vi "test_CCD_Setup_Testenvironment.vi"(6 "Delay between send and receive [ms]":i32=100, 8 "error in":errorcluster) -> (0 "error out":errorcluster, 2 "device open for communication?":bool, 3 "CCD out":refnum<class "CCD.lvclass">, 4 "Module Was Already Running?":bool)   [LabVIEW 2023]
uses:
  Classes/CCD/CCD.lvclass
  Libraries/DeviceManager/DeviceManager.lvlib
  <userlib>/_OpenG.lib/error/error.llb/openg_error.lvlib
panel:
  # "Connector Pane"
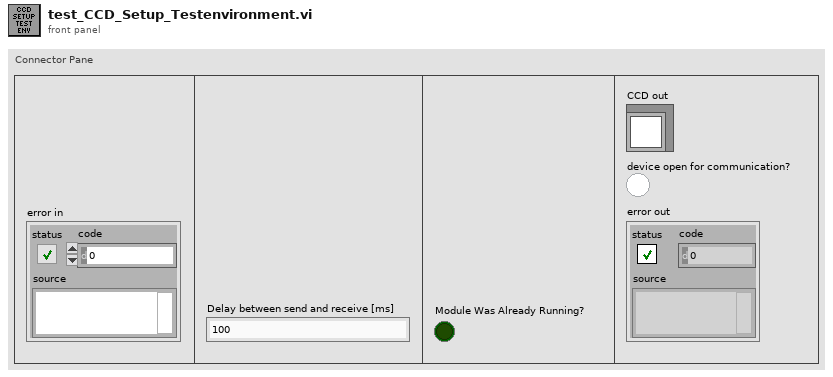
[diagram p1: front panel]
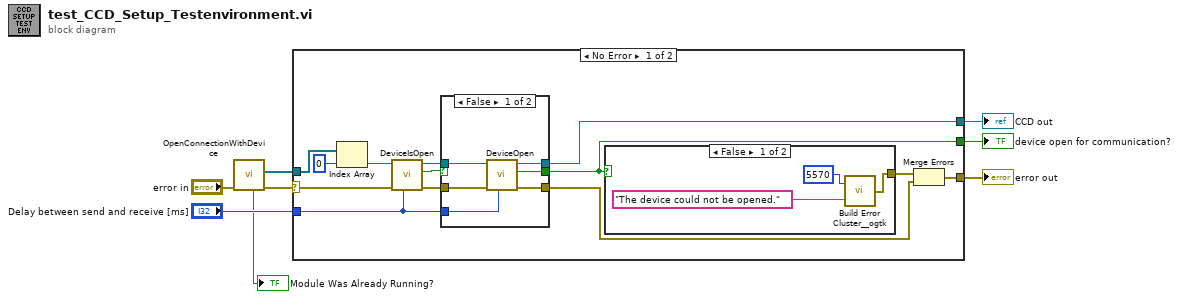
[diagram p0: block diagram]
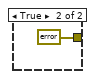
[diagram p3: hidden frame]
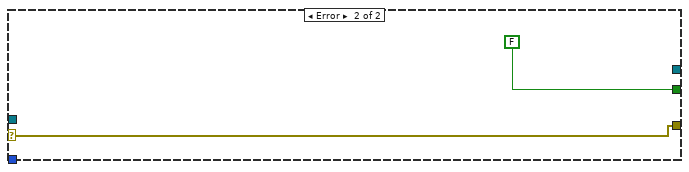
[diagram p4: hidden frame]
diagram:
  n1 = call "OpenConnectionWithDevice.vi"("error in"="error in") -> ("error out"=w3:errorcluster, "CCDs"=w4:refnum<class "CCD.lvclass">[], "Module Was Already Running?"=→"Module Was Already Running?":bool)  [unwired: 6 in, 2 out]
  n2 = case shown="No Error" w3 {
    selector: w3 -> [w11 w36]
    tunnel: w4 -> [w21 _]
    tunnel: [w19 w36] -> w7
    tunnel: [w12 FALSE ("CCD open for communication?")] -> w6
    tunnel: [w13 _] -> w5
    tunnel: "Delay between send and receive [ms]" -> [w9 _]
    frame No Error {
      n3 = Index Array(array=w21, index=0) -> (element=w14:refnum<class "CCD.lvclass">)
      n4 = call-dynamic "DeviceIsOpen.vi"("Delay between send and receive [ms]"=w9, "error in (no error)"=w11, "CCD in"=w14) -> ("error out"=w15:errorcluster, "device is open?"=w16:bool, "CCD out"=w17:refnum<class "CCD.lvclass">)  [unwired: 5 in, 1 out]
      n5 = case shown="False" w16 {
        selector: w16 -> [_ w28]
        tunnel: [w27 w28] -> w12
        tunnel: [w26 w29] -> w10
        tunnel: [w25 w30] -> w13
        tunnel: w15 -> [w24 w29]
        tunnel: w17 -> [w23 w30]
        tunnel: w9 -> [w22 _]
        frame False {
          n6 = call-dynamic "DeviceOpen.vi"("Delay between send and receive [ms]"=w22, "error in (no error)"=w24, "CCD in"=w23) -> ("error out"=w26:errorcluster, "device is open?"=w27:bool, "CCD out"=w25:refnum<class "CCD.lvclass">)  [unwired: 5 in, 1 out]
        }
        frame True {
        }
      }
      n7 = case shown="False" w12 {
        tunnel: [w32 errorcluster {"status"=FALSE, "code"=0, "source"=""} ("error in 2")] -> w18
        frame False {
          n8 = call <userlib>:"Build Error Cluster__ogtk.vi"("String to Prepend to source (\"\")"="The device could not be opened." ("String to Prepend to source (\"\")"), "code"=5570) -> ("error out"=w32:errorcluster)
        }
        frame True {
        }
      }
      n9 = Merge Errors(w18, w10) -> (w19:errorcluster)
    }
    frame Error {
    }
  }
  "error out" <- w7
  "device open for communication?" <- w6
  "CCD out" <- w5
